vi "LDO UI Setup Part 1.vi"(7 "Initialize? in":bool, 8 "error in (no error)":errorcluster, 11 "Queue in":refnum<queue>) -> (0 "error out":errorcluster, 3 "dup Message Queue":refnum<queue>)   [LabVIEW 2023]
uses:
  Message Queue/Message Cluster.ctl
  Message Queue/Enqueue Message (Single).vi
  Message Queue/Message Queue.lvlib
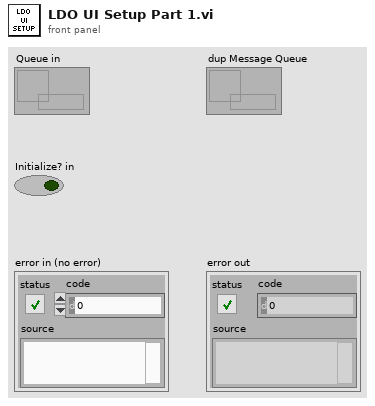
[diagram p1: front panel]
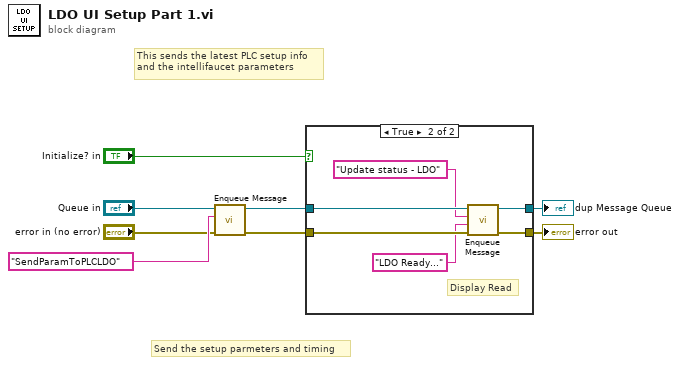
[diagram p0: block diagram]
diagram:
  # "This sends the latest PLC setup info\nand the intellifaucet parameters"
  # "Send the setup parmeters and timing"
  n1 = call-poly "Enqueue Message.vi"("error in (no error)"="error in (no error)", "Message"="SendParamToPLCLDO", "Message Queue"="Queue in") -> ("error out"=w2:errorcluster, "dup Message Queue"=w4:refnum<queue>)  [unwired: 7 in]
  n2 = case shown="True" "Initialize? in" {
    tunnel: w2 -> [w10 w16]
    tunnel: w4 -> [w9 w15]
    tunnel: [w10 w12] -> w7
    tunnel: [w9 w11] -> w1
    frame False {
    }
    frame True {
      # "Display Read"
      n3 = call-poly "Enqueue Message.vi"("error in (no error)"=w16, "Message Data"="LDO Ready..." ("Ready..."), "Message"="Update status - LDO", "Message Queue"=w15) -> ("error out"=w12:errorcluster, "dup Message Queue"=w11:refnum<queue>)  [unwired: 6 in]
    }
  }
  "error out" <- w7
  "dup Message Queue" <- w1
